vi "DeletedCommunity.vi"(11 "ProgramData":T1) -> ()   [LabVIEW 2018]
uses:
  ProductsCluster.ctl
panel:
  in  "OK Button":bool
  out "Usuniêty Produkt":T1
  # "Pomyœlnie usuniêto z bazy danych \n             nastêpuj¹cy produkt:"
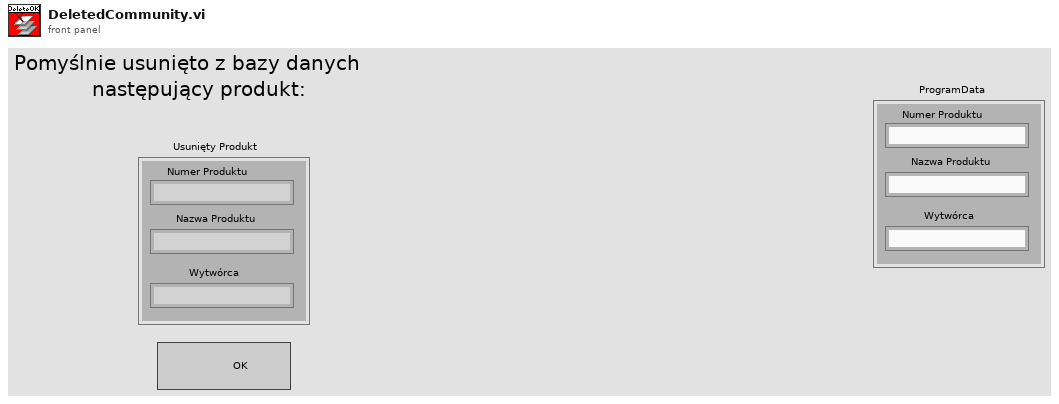
[diagram p1: front panel]
types:
  T1 = typedef "ProductsCluster.ctl" = cluster{"Numer Produktu":string, "Nazwa Produktu":string, "Wytwórca":string}
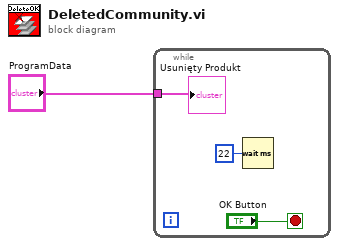
[diagram p0: block diagram]
diagram:
  n1 = while {
    tunnel: "ProgramData" -> [w4]
    stop <- "OK Button" stop-if-true
    n2 = Wait (ms)(milliseconds to wait=u32 22) -> ()  [unwired: 1 out]
    "Usuniêty Produkt" <- w4
  }
